vi "Reevaluate Target.vi"(9 "Delay Time (s)":dbl=1.0, 10 "error in (no error)":errorcluster) -> (2 "error out (no error)":errorcluster, 3 "What to do":string)   [LabVIEW 2015]
uses:
  Robot Global Data.vi
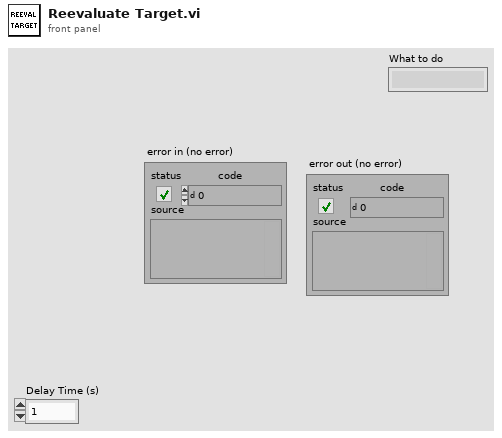
[diagram p1: front panel]
types:
  T1 = cluster{"Goal Left":dbl, "Goal Right":dbl, "Goal Width":dbl}
  T2 = typedef "Relevant Data.ctl" = cluster{"Area":dbl, "CH Area":dbl, "BR Width":dbl, "BR Height":dbl, "BR Left":dbl, "BR Right":dbl}
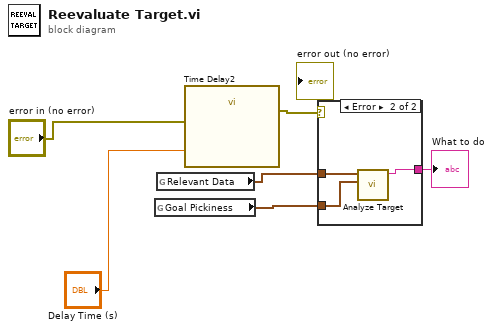
[diagram p0: block diagram]
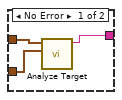
[diagram p2: hidden frame]
diagram:
  n1 = global read "Robot Global Data.vi" "Goal Pickiness"() -> (w2:T1)
  n2 = global read "Robot Global Data.vi" "Relevant Data"() -> (w3:T2[])
  n3 = call "Time Delay2"("error in (no error)"="error in (no error)", "Delay Time (s)"="Delay Time (s)") -> ("error out"=w4:errorcluster)  [unwired: 9 in]
  n4 = case shown="Error" w4 {
    tunnel: w3 -> [w9 w12]
    tunnel: w2 -> [w8 w11]
    tunnel: [w7 w10] -> w1
    frame No Error {
      n5 = call "Analyze Target.vi"("Goal Pickiness"=w8, "Relevant Data"=w9) -> ("What to do"=w7:string)  [unwired: 9 in]
    }
    frame Error {
      n6 = call "Analyze Target.vi"("Goal Pickiness"=w11, "Relevant Data"=w12) -> ("What to do"=w10:string)  [unwired: 9 in]
    }
  }
  "What to do" <- w1
